vi "E.ECU 19 (SubVI).vi"(6 "u(k)":dbl=30.0, 9 "C in":dbl[](array[numeric]), 10 "B in":dbl[](array[numeric]), 11 "A in":T1) -> (4 "Y(k)":dbl, 5 "X(t)":dbl[](array[numeric]))   [LabVIEW 2020]
uses:
  <vilib>/Analysis/Matrix/Datatypes/RealMatrix.ctl
  <vilib>/Analysis/baseanly.llb/A x Vector.vi
  <vilib>/Analysis/baseanly.llb/Real Dot Product.vi
  <menus>/Categories/IAControl Library/continuous linear.llb/Integrator (DBL Array).vi
  <vilib>/Analysis/NI_AALBase.lvlib
  <vilib>/Analysis/Matrix/NI_Matrix.lvlib
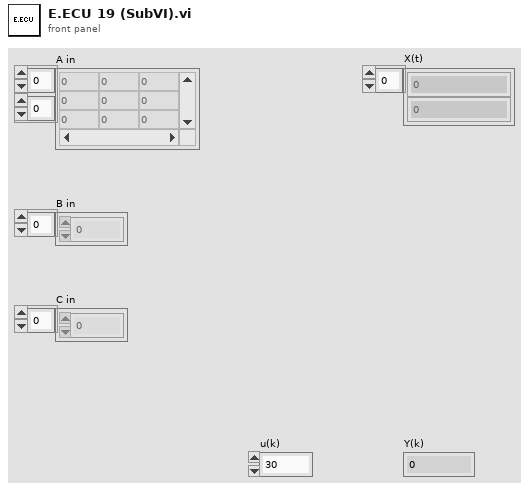
[diagram p1: front panel]
types:
  T1 = typedef "NI_Matrix.lvlib/RealMatrix.ctl" = dbl[][]
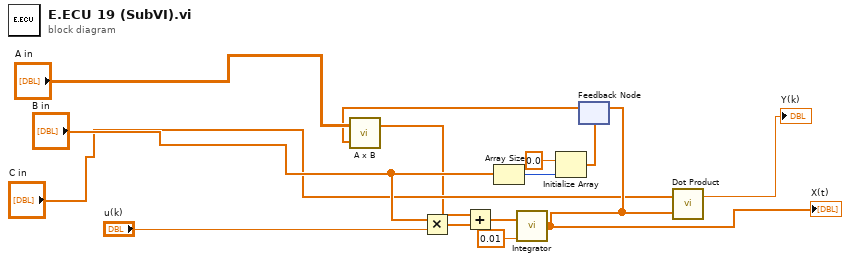
[diagram p0: block diagram]
diagram:
  n1 = Multiply(x="B in", y="u(k)") -> (x*y=w5:dbl[])
  n2 = Array Size(array="B in") -> (size(s)=w2:i32)
  n3 = Initialize Array(0.0 ("element"), w2) -> (w1:dbl[])
  n4 = feedback #1(w1) -> (w3:dbl[])
  n5 = call-poly <vilib>:"A x B.vi"("Vector"=w3, "A"="A in") -> ("A x Vector"=w6:dbl[])  [unwired: 1 out]
  n6 = Add ("Add.vi")(x=w6, y=w5) -> (x+y=w4:dbl[])
  n7 = call-poly <menus>:"Integrator.vi"("input points"=w4, "dt"=0.01) -> ("output points"=w14:dbl[])  [unwired: 13 in]
  "X(t)" <- w14
  n8 = feedback-in #1(w14) -> ()
  n9 = call-poly <vilib>:"Dot Product.vi"("Y Vector"=w14, "X Vector"="C in") -> ("X * Y"=→"Y(k)":dbl)  [unwired: 1 out]
